vi "Set Notifiers.vi"(8 "error in (no error)":errorcluster, 10 "Notifier":T1, 11 "Task Base in":refnum<class "Task Base.lvclass">) -> (0 "error out":errorcluster, 3 "Task Base out":refnum<class "Task Base.lvclass">)   [LabVIEW 2023, in "HAL GOOP4.lvlib" / "Task Base.lvclass"]
uses:
  Task Base.lvclass
  Task Base.lvclass/Task Base.ctl
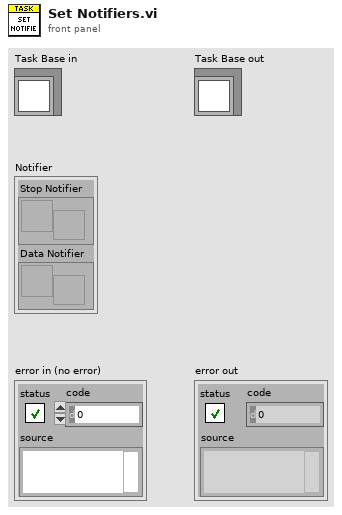
[diagram p1: front panel]
types:
  T1 = cluster{"Stop Notifier":refnum<notifier>, "Data Notifier":refnum<notifier>}
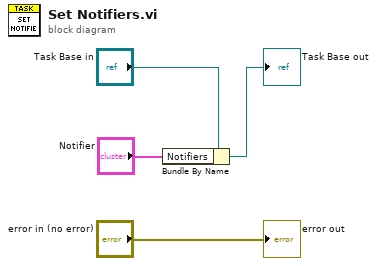
[diagram p0: block diagram]
diagram:
  n1 = Bundle By Name(cluster="Task Base in", "Notifiers"="Notifier") -> (→"Task Base out":refnum<class "Task Base.lvclass">)
  "error out" <- "error in (no error)"
